vi "orc-grey-rectangle.vi"(6 "Blue or Luma or Val or Inten Range":cluster{"Lower value":i32, "Upper value":i32}={"Lower value"=50, "Upper value"=104}, 8 "Image Src":T1, 9 "error in (no error)":errorcluster, 10 "Green or Sat Range":cluster{"Lower value":i32, "Upper value":i32}={"Lower value"=50, "Upper value"=84}, 11 "Red or Hue Range":cluster{"Lower value":i32, "Upper value":i32}={"Lower value"=50, "Upper value"=56}) -> (0 "error out":errorcluster, 1 "Image Out":T1(plugin-control), 2 "Particle Measurements (Pixels)":dbl[][](array[numeric]) format="%.2f", 4 "Particle Measurements (Real-World)":dbl[][](array[numeric]) format="%.2f")   [LabVIEW 2009]
uses:
  <vilib>/vision/Image Controls.llb/IMAQ Image.ctl
  <vilib>/vision/NI_Vision_Development_Module.lvlib
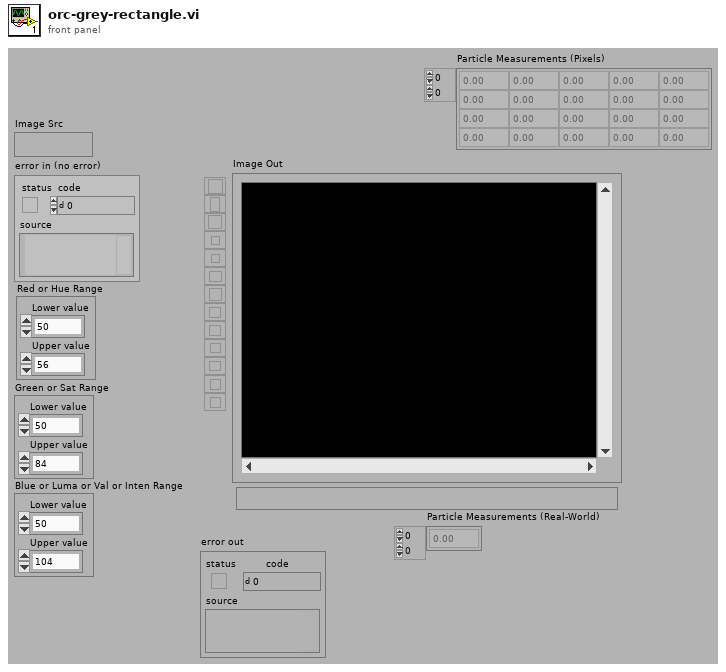
[diagram p1: front panel]
types:
  T1 = typedef "IMAQ Image.ctl" = refnum<image>
  T2 = typedef "Particle Parameters" = i32
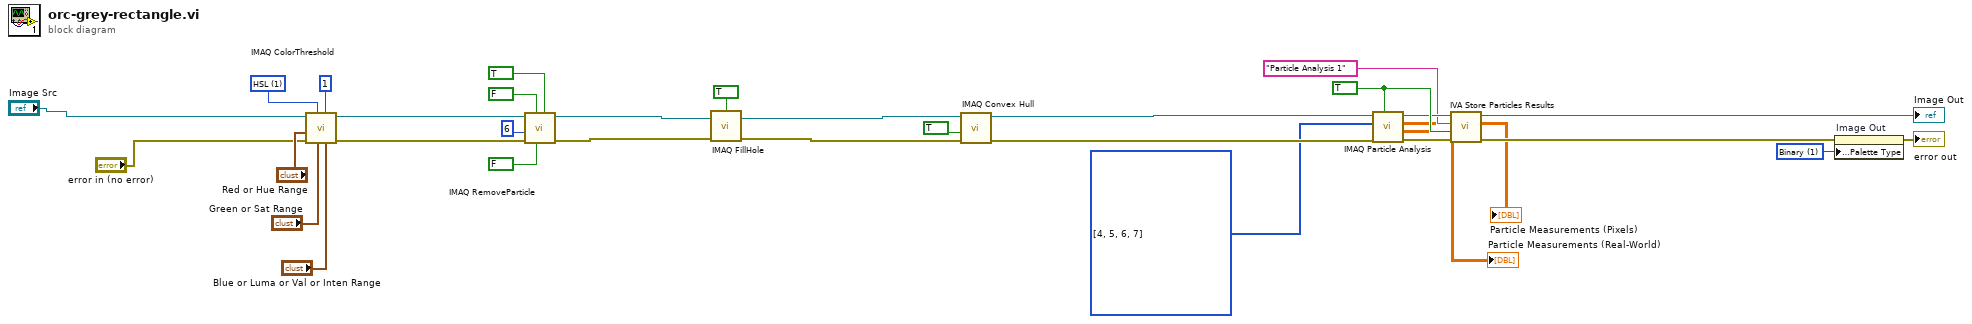
[diagram p0: block diagram]
diagram:
  w1 = T2[] [4, 5, 6, 7] items=["Center of Mass X", "Center of Mass Y", "First Pixel X", "First Pixel Y", "Bounding Rect Left", "Bounding Rect Top", "Bounding Rect Right", "Bounding Rect Bottom", "Max Feret Diameter Start X", "Max Feret Diameter Start Y", "Max Feret Diameter End X", "Max Feret Diameter End Y", "Max Horiz. Segment Length Left", "Max Horiz. Segment Length Right", "Max Horiz. Segment Length Row", "-", "Bounding Rect Width", "Bounding Rect Height", "Bounding Rect Diagonal", "Perimeter", "Convex Hull Perimeter", "Holes' Perimeter", "Max Feret Diameter", "Equivalent Ellipse Major Axis", "Equivalent Ellipse Minor Axis", "Equivalent Ellipse Minor Axis (Feret)", "Equivalent Rect Long Side", "Equivalent Rect Short Side", "Equivalent Rect Diagonal", "Equivalent Rect Short Side (Feret)", "Average Horiz. Segment Length", "Average Vert. Segment Length", "Hydraulic Radius", "Waddel Disk Diameter", "-", "Area", "Holes' Area", "Particle & Holes' Area", "Convex Hull Area", "Image Area", "-", "Number of Holes", "Number of Horiz. Segments", "Number of Vert. Segments", "-", "Orientation", "Max Feret Diameter Orientation", "-", "% Area/Image Area", "% Area/(Particle & Holes' Area)", "Ratio of Equivalent Ellipse Axes", "Ratio of Equivalent Rect Sides", "-", "Elongation Factor", "Compactness Factor", "Heywood Circularity Factor", "Type Factor", "-", "Sum X", "Sum Y", "Sum XX", "Sum XY", "Sum YY", "Sum XXX", "Sum XXY", "Sum XYY", "Sum YYY", "-", "Moment of Inertia XX", "Moment of Inertia XY", "Moment of Inertia YY", "Moment of Inertia XXX", "Moment of Inertia XXY", "Moment of Inertia XYY", "Moment of Inertia YYY", "Norm. Moment of Inertia XX", "Norm. Moment of Inertia XY", "Norm. Moment of Inertia YY", "Norm. Moment of Inertia XXX", "Norm. Moment of Inertia XXY", "Norm. Moment of Inertia XYY", "Norm. Moment of Inertia YYY", "Hu Moment 1", "Hu Moment 2", "Hu Moment 3", "Hu Moment 4", "Hu Moment 5", "Hu Moment 6", "Hu Moment 7"] ("Pixel Measurements")
  w7 = u32 1 items=["Grayscale", "Binary", "Gradient", "Rainbow", "Temperature", "User Defined"] ("Palette")
  w13 = TRUE ("Connectivity 4/8 (8)")
  w31 = u16 1 items=["RGB", "HSL", "HSV", "HSI"] ("Color Mode")
  n1 = call "IMAQ ColorThreshold"("Blue or Luma or Val or Inten Range"="Blue or Luma or Val or Inten Range", "Replace Value"=1, "Green or Sat Range"="Green or Sat Range", "Color Mode"=w31, "error in (no error)"="error in (no error)", "Red or Hue Range"="Red or Hue Range", "Image Src"="Image Src") -> ("error out"=w27:errorcluster, "Image Dst Out"=w22:T1)  [unwired: 1 in, 2 out]
  n2 = call "IMAQ RemoveParticle"("Connectivity 4/8 (8)"=TRUE, "Low Pass/High Pass (Low)"=FALSE, "Square/Hexa (Square)"=FALSE, "error in (no error)"=w27, "Number of Erosion"=6, "Image Src"=w22) -> ("error out"=w21:errorcluster, "Image Dst Out"=w19:T1)  [unwired: 1 in, 3 out]
  n3 = call "IMAQ FillHole"("error in (no error)"=w21, "Image Src"=w19, "Connectivity 4/8 (8)"=TRUE) -> ("error out"=w18:errorcluster, "Image Dst Out"=w17:T1)  [unwired: 1 in, 2 out]
  n4 = call "IMAQ Convex Hull"("error in (no error)"=w18, "Connectivity 4/8 (8)"=TRUE, "Image Src"=w17) -> ("error out"=w15:errorcluster, "Image Dst Out"=w14:T1)  [unwired: 1 in, 6 out]
  n5 = call "IMAQ Particle Analysis"("Connectivity 4/8 (8)"=w13, "error in (no error)"=w15, "Pixel Measurements"=w1, "Image"=w14) -> ("error out"=w10:errorcluster, "Particle Measurements (Real-World)"=→"Particle Measurements (Real-World)":dbl[][], "Particle Measurements (Pixels)"=→"Particle Measurements (Pixels)":dbl[][], "Image Out (duplicate)"=w12:T1)  [unwired: 1 in, 3 out]
  n6 = call <vilib>:"IVA Store Particles Results.vi"("error in (no error)"=w10, "Connectivity 4/8 (8)"=w13, "Step Name"="Particle Analysis 1", "Image in"=w12) -> ("error out"=w9:errorcluster, "Image dup"=→"Image Out":T1)  [unwired: 6 out]
  n7 = property on="Image Out" class="ImageControl"(error in=w9, "Palette:Palette Type"=w7) -> (error out=→"error out":errorcluster)  [unwired: 1 in, 1 out]
